vi "PM100D Simple Example.vi"() -> ()   [LabVIEW 2014]
doc: "This VI shows how to communicate with a PM100D optical power/energy meter with SCPI commands.\n- Initializing the instrument\n- Getting system info\n- Setting parameters\n- Measurement configuration\n- Measuring queue\n- Fetching and displaying a measurement value\n- Closing the application"
panel:
  out "Readout value":dbl format="%^#_9e"
  out "IDN String":string
  out "Sensor SN":string
  out "Sensor Name":string
  out "Sensor Flags":bool[](array[boolean])
  out "New":bool
  in  "Timeout [ms]":i32=1000
  in  "stop":bool
  in  "Readout Config":string(combo)="POW"
  out "Readout string":string
  out "Error log":string
  in  "Averaging Rate":i32=300
  # "1 Power Sensor"
  # "2 Energy Sensor"
  # "4"
  # "8"
  # "16 Response settable"
  # "32 Wavelength settable"
  # "64 Tau (time constant) settable"
  # "128"
  # "256 With temperature sensor"
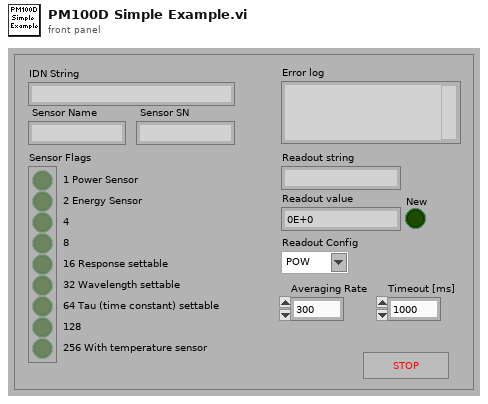
[diagram p1: front panel]
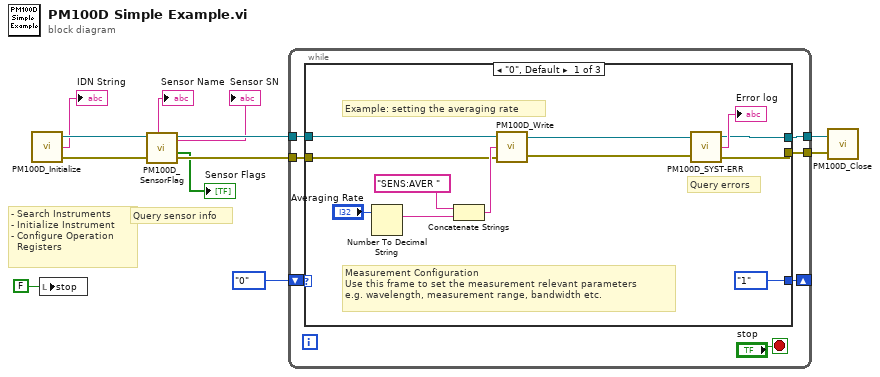
[diagram p0: block diagram]
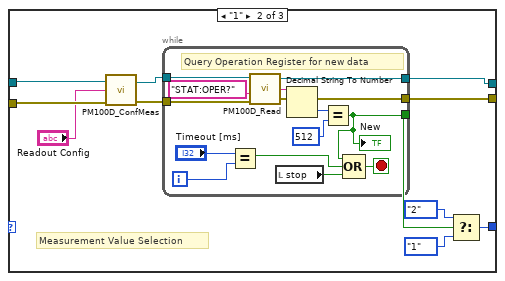
[diagram p2: hidden frame]
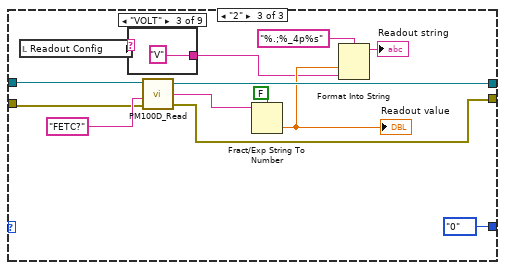
[diagram p3: hidden frame]
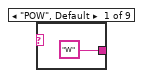
[diagram p4: hidden frame]
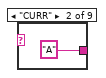
[diagram p5: hidden frame]
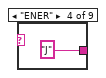
[diagram p6: hidden frame]
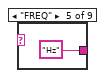
[diagram p7: hidden frame]
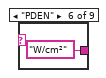
[diagram p8: hidden frame]
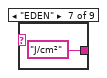
[diagram p9: hidden frame]
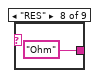
[diagram p10: hidden frame]
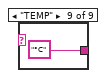
[diagram p11: hidden frame]
diagram:
  # "- Search Instruments\n- Initialize Instrument\n- Configure Operation\n  Registers"
  # "Query sensor info"
  n1 = call "PM100D_Initialize.vi"() -> ("error out"=w11:errorcluster, "Instrument"=→"IDN String":string, "VISA out"=w12:refnum<visa-resource-name>)  [unwired: 2 in, 1 out]
  n2 = local write "stop"(FALSE ("stop")) -> ()
  n3 = call "PM100D_SensorFlag.vi"("error in (no error)"=w11, "VISA in"=w12) -> ("error out"=w9:errorcluster, "flags"=→"Sensor Flags":bool[], "VISA out"=w10:refnum<visa-resource-name>, "sn"=→"Sensor SN":string, "name"=→"Sensor Name":string)  [unwired: 2 in, 3 out]
  n4 = while {
    tunnel: w10 -> [w19]
    tunnel: w9 -> [w18]
    shift-right: [w15] -> _
    shift-left: enum16{"0", "1", "2"}."0" -> [w16]
    tunnel: [w14] -> w3
    tunnel: [w13] -> w2
    stop <- "stop" stop-if-true
    n5 = case shown="\"0\", Default" w16 {
      tunnel: w19 -> [w28 w42 w67]
      tunnel: w18 -> [w23 w41 w66]
      tunnel: [enum16{"0", "1", "2"}."1" w36 enum16{"0", "1", "2"}."0"] -> w15
      tunnel: [w21 w38 w65] -> w14
      tunnel: [w20 w37 w57] -> w13
      frame "0", Default {
        # "Query errors"
        # "Example: setting the averaging rate"
        # "Measurement Configuration\nUse this frame to set the measurement relevant parameters\ne.g. wavelength, measurement range, bandwidth etc."
        n6 = Number To Decimal String(number="Averaging Rate") -> (decimal integer string=w30:string)  [unwired: 1 in]
        n7 = Concatenate Strings("SENS:AVER " ("string"), w30) -> (w27:string)
        n8 = call "PM100D_Write.vi"("error in (no error)"=w23, "Command"=w27, "VISA in"=w28) -> ("error out"=w24:errorcluster, "VISA out"=w26:refnum<visa-resource-name>)
        n9 = call "PM100D_SYST-ERR.vi"("error out 2"=w24, "VISA In"=w26) -> ("error out"=w20:errorcluster, "Error"=→"Error log":string, "VISA Out"=w21:refnum<visa-resource-name>)  [unwired: 1 in]
      }
      frame "1" {
        # "Measurement Value Selection"
        n10 = call "PM100D_ConfMeas.vi"("error in"=w41, "Conf:"="Readout Config", "VISA In"=w42) -> ("error out"=w39:errorcluster, "dup VISA session"=w40:refnum<visa-resource-name>)
        n11 = while {
          tunnel: w40 -> [w52]
          tunnel: w39 -> [w51]
          tunnel: [w50] -> w38
          tunnel: [w49] -> w37
          tunnel: [w43] -> w33
          i -> [w45]
          stop <- w47 stop-if-true
          # "Query Operation Register for new data"
          n12 = Equal?(x="Timeout [ms]", y=w45) -> (x = y?=w44:bool)
          n13 = call "PM100D_Read.vi"("error in (no error)"=w51, "Command"="STAT:OPER?", "VISA in"=w52) -> ("error out"=w49:errorcluster, "ReadValue"=w55:string, "VISA out"=w50:refnum<visa-resource-name>)  [unwired: 1 in]
          n14 = local read "stop"() -> (w48:bool)
          n15 = Decimal String To Number(string=w55) -> (number=w54:i32)  [unwired: 2 in, 1 out]
          n16 = Equal?(x=w54, y=512) -> (x = y?=w43:bool)
          "New" <- w43
          n17 = Compound Arithmetic op=OR(w43, w44, w48) -> (w47:bool)
        }
        n18 = Select(t=enum16{"0", "1", "2"}."2", s=w33, f=enum16{"0", "1", "2"}."1") -> (s? t:f=w36:enum16{"0", "1", "2"})
      }
      frame "2" {
        n19 = local read "Readout Config"() -> (w64:string)
        n20 = case shown="\"VOLT\"" w64 {
          tunnel: ["W" "A" "V" "J" "Hz" "W/cm²" "J/cm²" "Ohm" "°C"] -> w59
          frame "POW", Default {
          }
          frame "CURR" {
          }
          frame "VOLT" {
          }
          frame "ENER" {
          }
          frame "FREQ" {
          }
          frame "PDEN" {
          }
          frame "EDEN" {
          }
          frame "RES" {
          }
          frame "TEMP" {
          }
        }
        n21 = call "PM100D_Read.vi"("error in (no error)"=w66, "Command"="FETC?", "VISA in"=w67) -> ("error out"=w57:errorcluster, "ReadValue"=w63:string, "VISA out"=w65:refnum<visa-resource-name>)  [unwired: 1 in]
        n22 = Fract/Exp String To Number(use system decimal point (T)=FALSE, string=w63) -> (number=w60:dbl)  [unwired: 2 in, 1 out]
        "Readout value" <- w60
        n23 = Format Into String(format string="%.;%_4p%s", w60, w59) -> (resulting string=→"Readout string":string)  [unwired: 2 in, 1 out]
      }
    }
  }
  n24 = call "PM100D_Close.vi"("error in (no error)"=w2, "VISA resource name"=w3) -> ()  [unwired: 1 in, 1 out]
